vi "ScaleAndDrawImageInCenter.vi"(0 "reference in":refnum<class "LcPictureBox.lvclass">, 1 "Image":refnum<k24>, 5 "error in (no error)":errorcluster, 8 "SmoothingMode(AntiAlias)":T1=enum."AntiAlias") -> (14 "reference out":refnum<class "LcPictureBox.lvclass">, 15 "ImageOffset":cluster{"Numeric":dbl, "Numeric":dbl}, 16 "ZommScale":dbl, 19 "error out":errorcluster)   [LabVIEW 2020, in "LcPictureBox.lvclass"]
uses:
  LcPictureBox.lvclass
  System.Drawing
  SmoothingMode.ctl
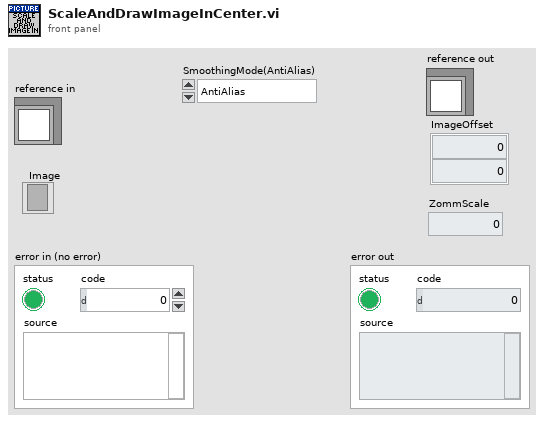
[diagram p1: front panel]
types:
  T1 = typedef "LcPictureBox.lvclass/SmoothingMode.ctl" = enum16{"None", "HighSpeed", "HighQuality", "AntiAlias"}
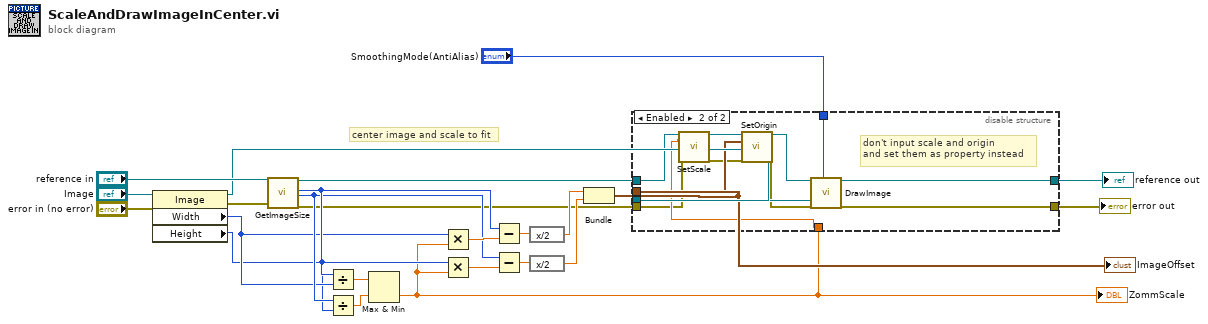
[diagram p0: block diagram]
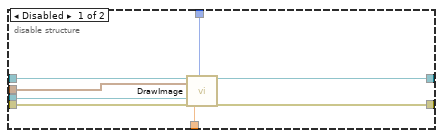
[diagram p2: hidden frame]
diagram:
  # "center image and scale to fit"
  n1 = property class="Image"(reference="Image", error in="error in (no error)") -> (reference out=w6:refnum<k24>, error out=w16:errorcluster, "Width"=w9:i32, "Height"=w8:i32)
  n2 = call-dynamic "GetImageSize.vi"("reference in"="reference in", "error in (no error)"=w16) -> ("reference out"=w15:refnum<class "LcPictureBox.lvclass">, "Width"=w12:i32, "Height"=w11:i32, "error out"=w1:errorcluster)  [unwired: 14 in]
  n3 = Divide(x=w12, y=w9) -> (x/y=w17:dbl)
  n4 = Divide(x=w11, y=w8) -> (x/y=w18:dbl)
  n5 = Max & Min(x=w17, y=w18) -> (min(x,y)=w2:dbl)  [unwired: 1 out]
  "ZommScale" <- w2
  n6 = Multiply(x=w9, y=w2) -> (x*y=w22:dbl)
  n7 = Multiply(x=w8, y=w2) -> (x*y=w21:dbl)
  n8 = Subtract(x=w12, y=w22) -> (x-y=w19:dbl)
  n9 = Subtract(x=w11, y=w21) -> (x-y=w20:dbl)
  n10 = expression code="x/2"(w19) -> (w23:dbl)
  n11 = expression code="x/2"(w20) -> (w24:dbl)
  n12 = Bundle(w23, w24) -> (w3:cluster{dbl, dbl})  [unwired: 1 in]
  "ImageOffset" <- w3
  n13 = disable-structure shown="Enabled" {
    disable-tunnel: w15 -> [w32 w37]
    disable-tunnel: [w31 w44] -> w10
    disable-tunnel: w6 -> [w30 w43]
    disable-tunnel: [w29 w42] -> w5
    disable-tunnel: "SmoothingMode(AntiAlias)" -> [w28 w41]
    disable-tunnel: w3 -> [w27 w39]
    disable-tunnel: w1 -> [w26 w34]
    disable-tunnel: w2 -> [w25 w35]
    frame Disabled {
      n14 = call-dynamic "DrawImage.vi"("reference in"=w32, "UpperLeftCorner(0,0)"=w27, "Image"=w30, "Error In"=w26, "ScaleFactor(1)"=w25, "SmoothingMode(AntiAlias)"=w28) -> ("reference out"=w29:refnum<class "LcPictureBox.lvclass">, "Error Out"=w31:errorcluster)  [unwired: 12 in]
    }
    frame Enabled {
      # "don't input scale and origin\nand set them as property instead"
      n15 = call-dynamic "SetScale.vi"("reference in"=w37, "ScaleFactor"=w35, "Error In"=w34) -> ("reference out"=w40:refnum<class "LcPictureBox.lvclass">, "Error Out"=w36:errorcluster)  [unwired: 15 in]
      n16 = call-dynamic "SetOrigin.vi"("reference in"=w40, "Origin"=w39, "Error In"=w36) -> ("reference out"=w38:refnum<class "LcPictureBox.lvclass">, "Error Out"=w33:errorcluster)  [unwired: 15 in]
      n17 = call-dynamic "DrawImage.vi"("reference in"=w38, "Image"=w43, "Error In"=w33, "SmoothingMode(AntiAlias)"=w41) -> ("reference out"=w42:refnum<class "LcPictureBox.lvclass">, "Error Out"=w44:errorcluster)  [unwired: 14 in]
    }
  }
  "error out" <- w10
  "reference out" <- w5
